vi "trigger.vi"(0 "triggerReadout":u16) -> (14 "triggered":bool)   [LabVIEW 2014]
uses:
  triggerGlobalVars.vi
  Sequencer/sequencerGlobVars.vi
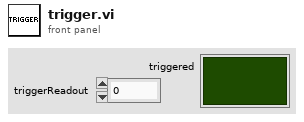
[diagram p1: front panel]
types:
  T1 = typedef "selectTrigger.ctl" = enum8{"Ext0", "Ext1", "Ext2", "Ext3", "Ext4", "Ext5", "Ext6", "Ext7", "Int0", "Int1", "Int2", "Int3", "Int4", "Int5", "Int6", "Int7"}
  T2 = typedef "triggerTypes.ctl" = enum16{"noTrigger", "singleHitDelay", "singleHit", "software", "sweep"}
  T3 = typedef "triggerEdge.ctl" = enum8{"either", "false-true", "true-false"}
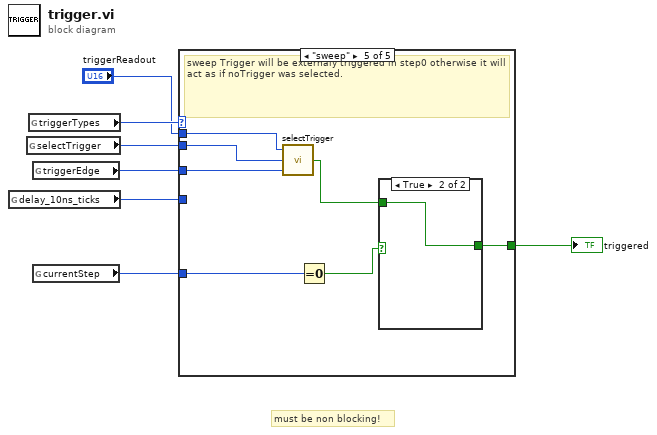
[diagram p0: block diagram]
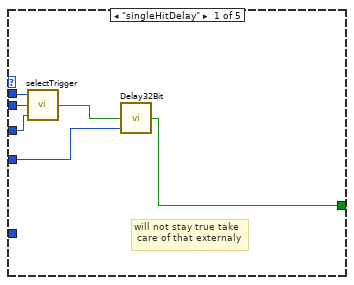
[diagram p2: hidden frame]
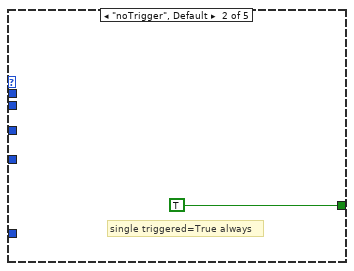
[diagram p3: hidden frame]
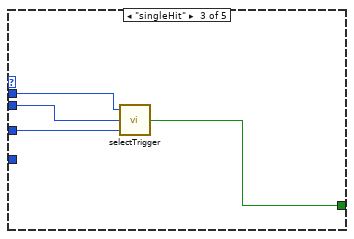
[diagram p4: hidden frame]
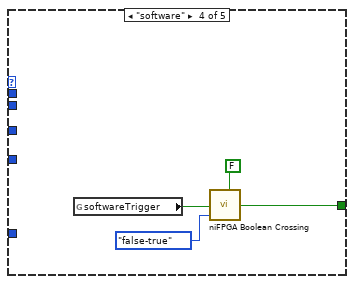
[diagram p5: hidden frame]
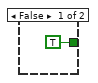
[diagram p6: hidden frame]
diagram:
  # "must be non blocking!"
  n1 = global read "triggerGlobalVars.vi" "delay_10ns_ticks"() -> (w4:u32)
  n2 = global read "triggerGlobalVars.vi" "selectTrigger"() -> (w5:T1)
  n3 = global read "triggerGlobalVars.vi" "triggerTypes"() -> (w6:T2)
  n4 = global read "triggerGlobalVars.vi" "triggerEdge"() -> (w3:T3)
  n5 = global read "sequencerGlobVars.vi" "currentStep"() -> (w2:i32)
  n6 = case shown="\"sweep\"" w6 {
    tunnel: w5 -> [w13 _ w18 _ w29]
    tunnel: w4 -> [w11 _ _ _ _]
    tunnel: [w10 TRUE w16 w22 w24] -> w7
    tunnel: w3 -> [w9 _ w17 _ w28]
    tunnel: w2 -> [_ _ _ _ w27]
    tunnel: "triggerReadout" -> [w8 _ w15 _ w23]
    frame "singleHitDelay" {
      # "will not stay true take\n care of that externaly"
      n7 = call "selectTrigger.vi"("triggerEdge"=w9, "MCSSelectTrigger"=w13, "triggerReadout"=w8) -> ("fired"=w12:bool)  [unwired: 2 in]
      n8 = call "Delay32Bit.vi"("delay(ticks)"=w11, "In"=w12) -> ("Out"=w10:bool)  [unwired: 3 in]
    }
    frame "noTrigger", Default {
      # "single triggered=True always"
    }
    frame "singleHit" {
      n9 = call "selectTrigger.vi"("triggerEdge"=w17, "MCSSelectTrigger"=w18, "triggerReadout"=w15) -> ("fired"=w16:bool)  [unwired: 2 in]
    }
    frame "software" {
      n10 = global read "triggerGlobalVars.vi" "softwareTrigger"() -> (w21:bool)
      n11 = call <vilib>:"niFPGA Boolean Crossing.vi"("input"=w21, "direction"=enum8{"either", "false-true", "true-false"}."false-true", "initialize"=FALSE) -> ("crossing"=w22:bool)  [unwired: 6 in]
    }
    frame "sweep" {
      # "sweep Trigger will be externaly triggered in step0 otherwise it will act as if noTrigger was selected."
      n12 = call "selectTrigger.vi"("triggerEdge"=w28, "MCSSelectTrigger"=w29, "triggerReadout"=w23) -> ("fired"=w25:bool)  [unwired: 2 in]
      n13 = Equal To 0?(x=w27) -> (x = 0?=w26:bool)
      n14 = case shown="True" w26 {
        tunnel: w25 -> [_ w31]
        tunnel: [TRUE ("fired") w31] -> w24
        frame False {
        }
        frame True {
        }
      }
    }
  }
  "triggered" <- w7
